vi "BLMultiplotPrepare.vi"(6 "HeightAxisBounds":T1, 7 "ProfileFilename":string, 9 "YaxisMapping":enum8{"Lin", "Log"}(ring), 10 "jitterFraction":dbl) -> (3 "gnuplotOut":string)   [LabVIEW 2014]
uses:
  minAndMax.ctl
  AutoManualNumber.ctl
  margins.ctl
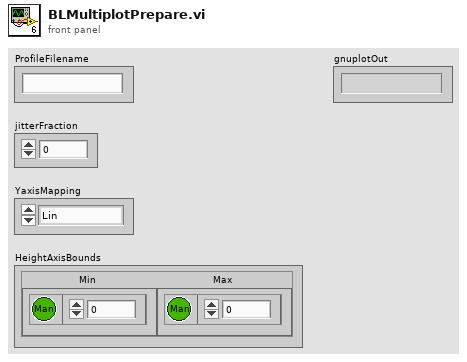
[diagram p1: front panel]
types:
  T1 = typedef "minAndMax.ctl" = cluster{"Min":T2, "Max":T2}
  T2 = typedef "AutoManualNumber.ctl" = cluster{"Auto":bool, "Value":dbl}
  T3 = typedef "margins.ctl" = cluster{"Top":dbl, "Bottom":dbl, "Left":dbl, "Right":dbl}
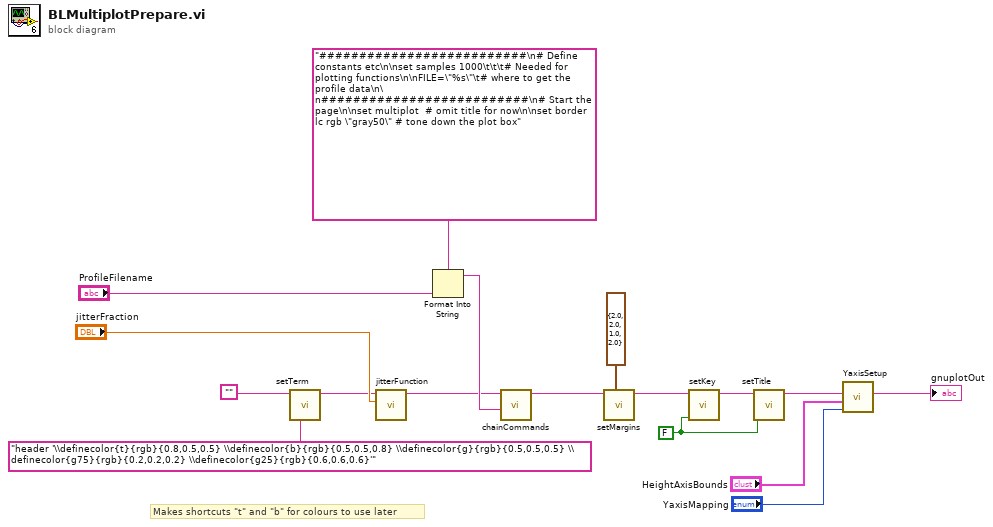
[diagram p0: block diagram]
diagram:
  w12 = FALSE ("Set?")
  # "Makes shortcuts \"t\" and \"b\" for colours to use later"
  n1 = call "setTerm.vi"("Additional Terminal Options"="header '\\definecolor{t}{rgb}{0.8,0.5,0.5} \\definecolor{b}{rgb}{0.5,0.5,0.8} \\definecolor{g}{rgb}{0.5,0.5,0.5} \\definecolor{g75}{rgb}{0.2,0.2,0.2} \\definecolor{g25}{rgb}{0.6,0.6,0.6}'", "String in"="") -> ("String out"=w2:string)  [unwired: 8 in, 1 out]
  n2 = call "jitterFunction.vi"("jitterFraction"="jitterFraction", "String in"=w2) -> ("String out"=w7:string)  [unwired: 8 in, 1 out]
  n3 = Format Into String(format string="##########################\n# Define constants etc\n\nset samples 1000\t\t\t# Needed for plotting functions\n\nFILE=\"%s\"\t# where to get the profile data\n\n##########################\n# Start the page\n\nset multiplot  # omit title for now\n\nset border lc rgb \"gray50\" # tone down the plot box" ("Command"), "ProfileFilename") -> (resulting string=w10:string)  [unwired: 2 in, 1 out]
  n4 = call "chainCommands.vi"("Command"=w10, "StringIn"=w7) -> ("StringOut"=w8:string)  [unwired: 9 in]
  n5 = call "setMargins.vi"("Margins"=T3 {"Top"=2.0, "Bottom"=2.0, "Left"=1.0, "Right"=2.0}, "String in"=w8) -> ("String out"=w5:string)  [unwired: 8 in, 1 out]
  n6 = call "setKey.vi"("Set?"=w12, "String in"=w5) -> ("String out"=w6:string)  [unwired: 8 in, 1 out]
  n7 = call "setTitle.vi"("Set?"=w12, "String in"=w6) -> ("String out"=w13:string)  [unwired: 8 in, 1 out]
  n8 = call "YaxisSetup.vi"("Mapping"="YaxisMapping", "HeightAxisBounds"="HeightAxisBounds", "gnuplotIn"=w13) -> ("gnuplotOut"=→"gnuplotOut":string)  [unwired: 8 in]
